vi "Create meas file with date.vi"(5 "Start point":dbl, 6 "Ambient T":dbl, 7 "End point":dbl, 8 "error in (no error)":errorcluster, 9 "Temperature setpoints":dbl[](array[numeric]), 10 "Sensor 2 name":string, 11 "Sensor 1 name":string) -> (0 "error out":errorcluster, 3 "tdms file out":refnum<k34>)   [LabVIEW 2021]
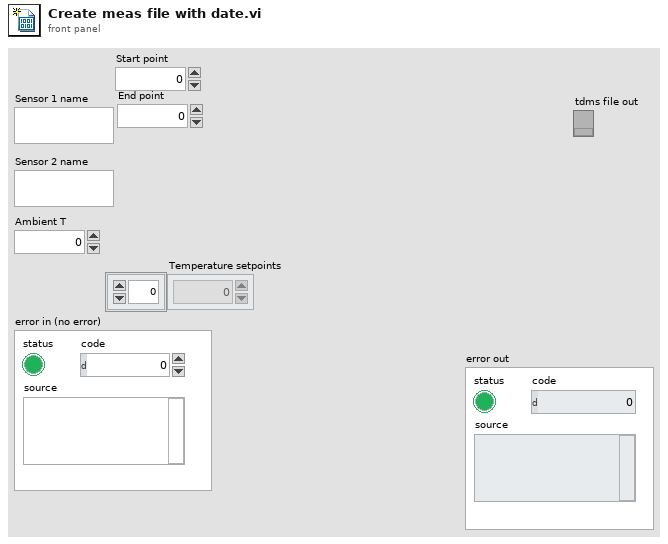
[diagram p1: front panel]
types:
  T1 = enum16{"open", "open or create", "create or replace", "create", "open (read-only)"}
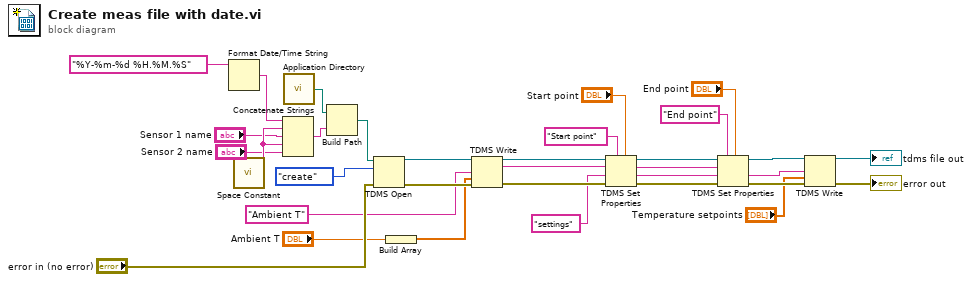
[diagram p0: block diagram]
diagram:
  n1 = Format Date/Time String(time format string (%c)="%Y-%m-%d %H.%M.%S") -> (date/time string=w15:string)  [unwired: 2 in]
  n2 = call <vilib>:"Space Constant.vi"() -> ("String"=w23:string)
  n3 = Concatenate Strings(w15, w23, "Sensor 1 name", w23, "Sensor 2 name") -> (w19:string)
  n4 = call <vilib>:"Application Directory.vi"() -> ("Application Directory"=w18:path)
  n5 = Build Path(base path=w18, name or relative path=w19) -> (appended path=w20:path)
  n6 = TDMS Open(8:"error in (no error)", 10:T1."create" ("operation (0:open)"), 11:w20) -> (0:w30:errorcluster, 3:w24:refnum<k34>)  [unwired: 4 in]
  n7 = Build Array("Ambient T") -> (w5:dbl[])
  n8 = TDMS Write(0:w24, 7:"Ambient T" ("channel name(s) in (Untitled)"), 9:w5, 11:w30) -> (4:w25:refnum<k34>, 6:w2:string, 15:w29:errorcluster)  [unwired: 2 in, 1 out]
  n9 = TDMS Set Properties(5:"Start point", 7:"Start point" ("channel name(s) in (Untitled)"), 8:w29, 9:"settings" ("channel name(s) in (Untitled)"), 10:w2, 11:w25) -> (0:w28:errorcluster, 1:w8:string, 2:w1:string, 3:w26:refnum<k34>)
  n10 = TDMS Set Properties(5:"End point", 7:"End point" ("channel name(s) in (Untitled)"), 8:w28, 9:w8, 10:w1, 11:w26) -> (0:w31:errorcluster, 1:w6:string, 3:w27:refnum<k34>)  [unwired: 1 out]
  n11 = TDMS Write(0:w27, 7:w6, 9:"Temperature setpoints", 11:w31) -> (4:→"tdms file out":refnum<k34>, 15:→"error out":errorcluster)  [unwired: 2 in, 2 out]
